vi "Data_Write.vi"(0 "Command List":T1, 1 "name":string, 2 "Data":string, 3 "error initialize":errorcluster) -> (6 "path":path, 7 "filename":string, 9 "error out":errorcluster)   [LabVIEW 2015]
uses:
  Data Write Control.ctl
panel:
  out "cancelled 2":bool
  out "cancelled":bool
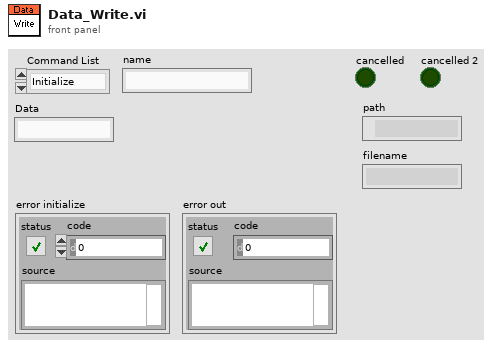
[diagram p1: front panel]
types:
  T1 = typedef "Data Write Control.ctl" = enum16{"Initialize", "Read", "Write", "Close"}
  T2 = enum16{"open", "replace", "create", "open or create", "replace or create", "replace or create with confirmation"}
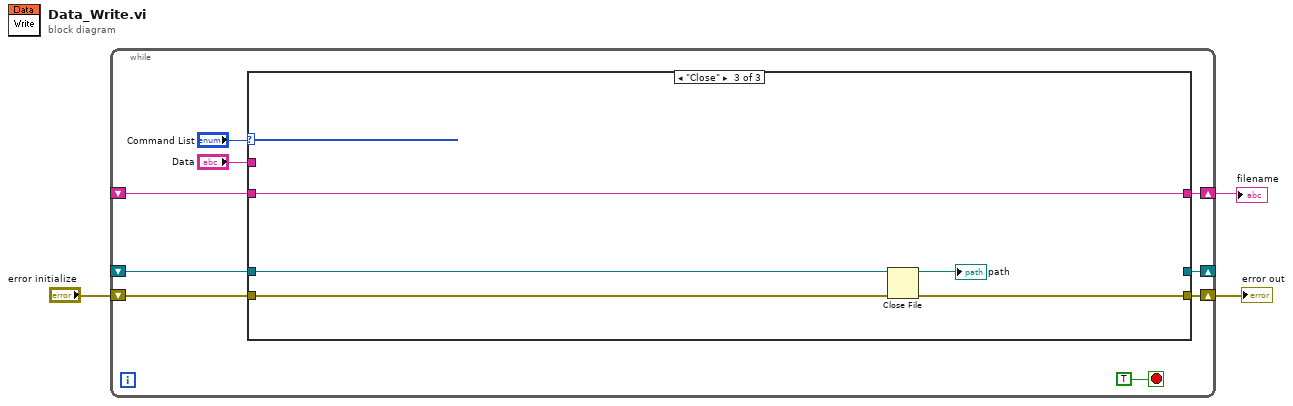
[diagram p0: block diagram]
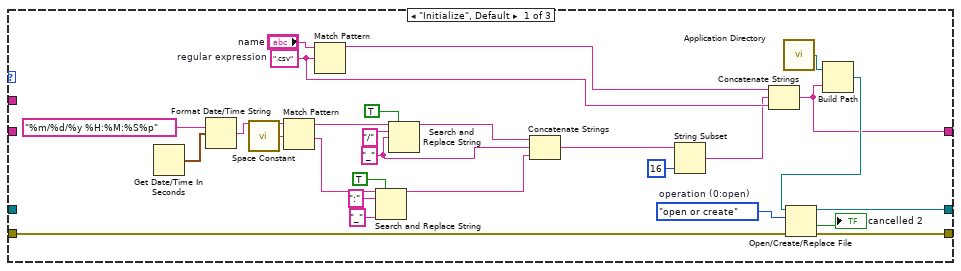
[diagram p2: hidden frame]
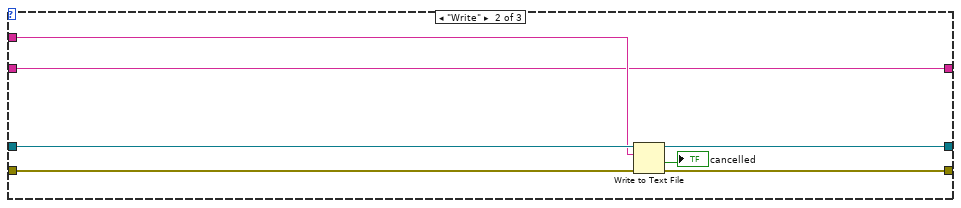
[diagram p3: hidden frame]
diagram:
  n1 = while {
    shift-right: [w9] -> w3
    shift-left: "error initialize" -> [w8]
    shift-right: [w7] -> _
    shift-left: _ -> [w6]
    shift-right: [w5] -> w1
    shift-left: _ -> [w4]
    stop <- TRUE stop-if-true
    n2 = case shown="\"Close\"" "Command List" {
      tunnel: "Data" -> [_ w43 _]
      tunnel: [w40 w47 w52] -> w9
      tunnel: w8 -> [w39 w46 w51]
      tunnel: [w38 w45 _] -> w7
      tunnel: w6 -> [_ w44 w50]
      tunnel: [w13 w41 w48] -> w5
      tunnel: w4 -> [_ w41 w48]
      frame "Initialize", Default {
        w14 = "_" ("replace string (\"\")")
        w17 = ".csv"  # regular expression
        w35 = T2."open or create"  # operation (0:open)
        n3 = Get Date/Time In Seconds() -> (seconds since 1Jan1904=w33:timestamp)
        n4 = Format Date/Time String(time format string (%c)="%m/%d/%y %H:%M:%S%p", seconds (now)=w33) -> (date/time string=w30:string)  [unwired: 1 in]
        n5 = call <vilib>:"Space Constant.vi"() -> ("String"=w29:string)
        n6 = Match Pattern(string=w30, regular expression=w29) -> (before substring=w28:string, after substring=w26:string)  [unwired: 1 in, 2 out]
        n7 = Match Pattern(string="name", regular expression=w17) -> (before substring=w15:string)  [unwired: 1 in, 3 out]
        n8 = Search and Replace String(replace all?=TRUE ("replace all? (F)"), input string=w26, search string=":", replace string="_" ("replace string (\"\")")) -> (result string=w22:string)  [unwired: 4 in, 3 out]
        n9 = Search and Replace String(replace all?=TRUE ("replace all? (F)"), input string=w28, search string="/", replace string=w14) -> (result string=w23:string)  [unwired: 4 in, 3 out]
        n10 = Concatenate Strings "Concatenate Strings"(w23, w14, w22) -> (w19:string)
        n11 = String Subset(string=w19, length (rest)=16 ("length (rest)")) -> (substring=w16:string)  [unwired: 1 in]
        n12 = Concatenate Strings "Concatenate Strings"(w15, w16, w17) -> (w13:string)
        n13 = call <vilib>:"Application Directory.vi"() -> ("Application Directory"=w34:path)
        n14 = Build Path(base path=w34, name or relative path=w13) -> (appended path=w37:path)
        n15 = Open/Create/Replace File(file path (use dialog)=w37, error in=w39, operation (0:open)=w35) -> (refnum out=w38:refnum<file>, cancelled=→"cancelled 2":bool, error out=w40:errorcluster)  [unwired: 3 in]
      }
      frame "Write" {
        n16 = Write to Text File(file (use dialog)=w44, text=w43, error in=w46) -> (refnum out=w45:refnum<file>, cancelled=→"cancelled":bool, error out=w47:errorcluster)  [unwired: 1 in]
      }
      frame "Close" {
        n17 = Close File(refnum=w50, error in=w51) -> (path=→"path":path, error out=w52:errorcluster)
      }
    }
  }
  "error out" <- w3
  "filename" <- w1
